vi "displayConfigurableElements.vi"(11 "ConfigurationThisComponent in":refnum<class "ConfigurationTestParameters.lvclass">) -> (3 "ConfigurationThisComponent out":refnum<class "ConfigurationTestParameters.lvclass">)   [LabVIEW 2015, in "ConfigurationTestParameters.lvclass"]
uses:
  ConfigurationTestParameters.lvclass
  Configuration/TestParameters.ctl
  Configuration/CycleProfileConfig.ctl
  <userlib>/Common/Log/Config/Log.ctl
  Typedefs/Pressure Servo Settings.ctl
  Typedefs/DAC Settings.ctl
  <userlib>/Common/Log/Log.lvlib
  Typedefs/FAMTTypedefs.lvlib
panel:
  in  "ctrlRefArrayUsrEvnt":refnum<user-event>
  in  "ConfigTab":T1(tab)
  in  "TestParameters":T2 {"Cycle profile"."Pause After" min=0.0 max=600.0 format="%.1f"; "Cycle profile"."Force Setpoint" min=-888.0 max=888.0 format="%.1f"; "Number of cycles for complete test" min=1}
  in  "TestDataLog":T4={"Log Directory"=path "", "Log Filename Base"="", "Max records per file"=1000, "Comment"=""} {"Max records per file" min=100 max=1000000}
  in  "StiffnessLog":T4={"Log Directory"=path "", "Log Filename Base"="", "Max records per file"=1000, "Comment"=""} {"Max records per file" min=100 max=1000000}
  in  "Pressure Servo Settings":T5={"Center Point"=413685.4733709468, "Area"=0.004536, "PA to PSI"=0.000145038, "Servo 1 DAC Channel"=1, "Servo 2 DAC Channel"=2} {"Servo 2 DAC Channel" min=1 max=4 step=1; "Servo 1 DAC Channel" min=1 max=4 step=1; "PA to PSI" format="%.9f"; "Area" format="%.9f"; "Center Point" format="%.3f"}
  in  "DAC Settings":T6={"Voltage Reference"=4.096, "Min Counts"=0, "Max Counts"=65535} {"Voltage Reference" format="%.3f"}
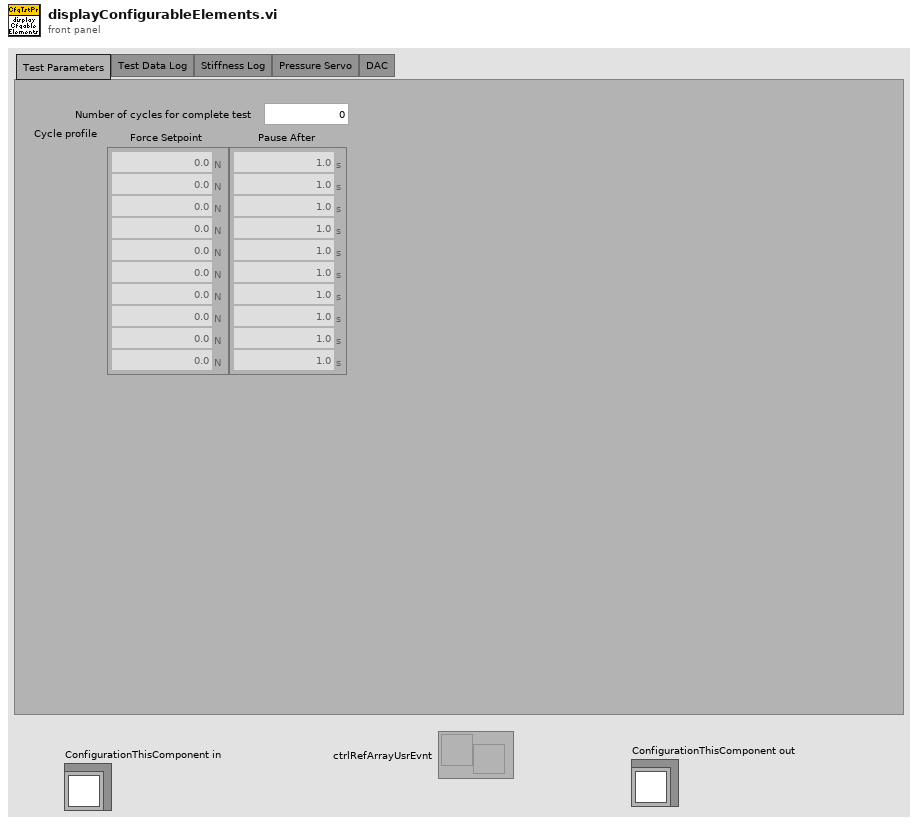
[diagram p1: front panel]
types:
  T1 = enum32{"Test Parameters", "Test Data Log", "Stiffness Log", "Pressure Servo", "DAC"}
  T2 = typedef "TestParameters.ctl" = cluster{"Number of cycles for complete test":u32, "Cycle profile":T3}
  T3 = typedef "CycleProfileConfig.ctl" = cluster{"Force Setpoint":dbl[unit][], "Pause After":dbl[unit][]}
  T4 = typedef "Log.lvlib/Log.ctl" = cluster{"Log Directory":path, "Log Filename Base":string, "Max records per file":u32, "Comment":string}
  T5 = typedef "FAMTTypedefs.lvlib/Pressure Servo Settings.ctl" = cluster{"Center Point":dbl[unit], "Area":dbl, "PA to PSI":dbl, "Servo 1 DAC Channel":u8, "Servo 2 DAC Channel":u8}
  T6 = typedef "FAMTTypedefs.lvlib/DAC Settings.ctl" = cluster{"Voltage Reference":dbl[unit], "Min Counts":i32, "Max Counts":i32}
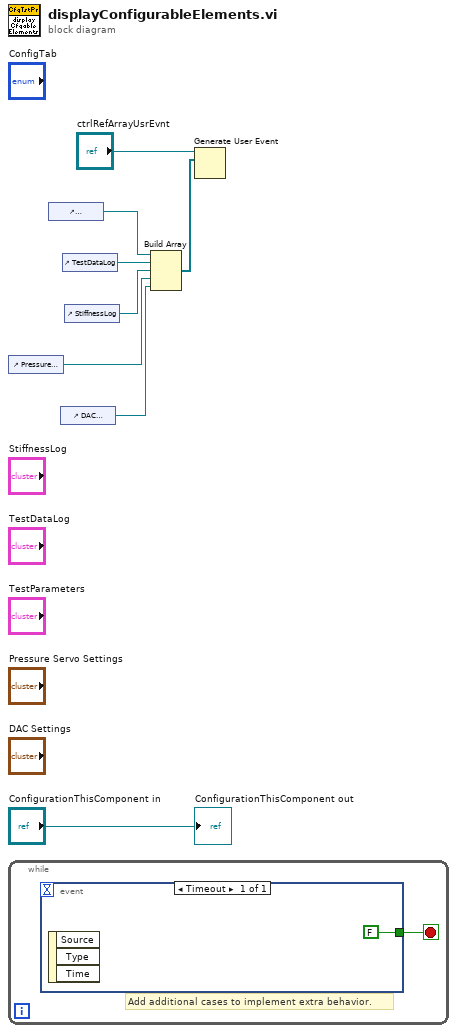
[diagram p0: block diagram]
diagram:
  n1 = control-ref of="Pressure Servo Settings"() -> (w2:refnum<vi>)
  n2 = while {
    stop <- w9 stop-if-true
    # "Add additional cases to implement extra behavior."
    n3 = event shown="[0] Timeout" {
      selector: _ -> [_]
      dyn-events: _ -> [_]
      timeout: _ -> [_]
      tunnel: [FALSE] -> w9
      event Timeout {
        n4 = event-data() -> ()  [unwired: 1 in, 3 out]
      }
    }
  }
  n5 = control-ref of="TestParameters"() -> (w6:refnum<vi>)
  n6 = control-ref of="DAC Settings"() -> (w1:refnum<vi>)
  n7 = control-ref of="TestDataLog"() -> (w4:refnum<vi>)
  n8 = control-ref of="StiffnessLog"() -> (w3:refnum<vi>)
  n9 = Build Array(w6, w4, w3, w2, w1) -> (w5:refnum<vi>[])
  n10 = Generate User Event(user event="ctrlRefArrayUsrEvnt", event data cluster=w5) -> ()  [unwired: 2 in, 2 out]
  "ConfigurationThisComponent out" <- "ConfigurationThisComponent in"
